vi "get_env_variable.vi"(3 "Environment Variable Name":string) -> (0 "error out":errorcluster, 1 "Value":string)   [LabVIEW 2020]
uses:
  <vilib>/Utility/config.llb/Read Key (String).vi
  <vilib>/Utility/config.llb/NI_LVConfig.lvlib
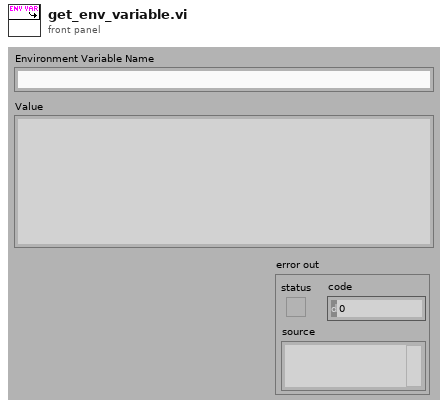
[diagram p1: front panel]
types:
  T1 = typedef "NI_LVConfig.lvlib/Config Data RefNum.ctl" = refnum<k1>
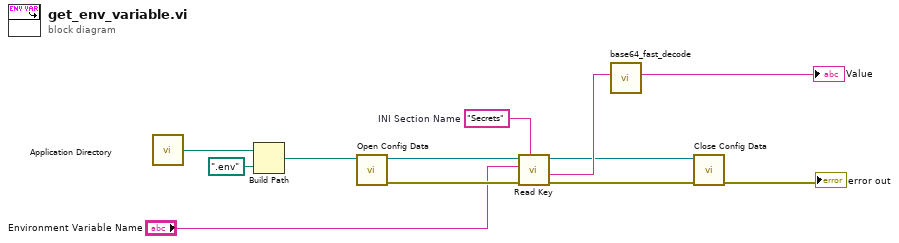
[diagram p0: block diagram]
diagram:
  w9 = "Secrets"  # INI Section Name
  n1 = call <vilib>:"Application Directory.vi"() -> ("Application Directory"=w12:path)
  n2 = Build Path(base path=w12, name or relative path=path ".env") -> (appended path=w10:path)
  n3 = call <vilib>:"Open Config Data.vi"("configuration file path"=w10) -> ("error out"=w8:errorcluster, "refnum"=w7:T1)  [unwired: 8 in, 1 out]
  n4 = call-poly <vilib>:"Read Key.vi"("section"=w9, "error in (no error)"=w8, "key"="Environment Variable Name", "refnum"=w7) -> ("error out"=w3:errorcluster, "value"=w5:string, "refnum out"=w2:T1)  [unwired: 4 in, 1 out]
  n5 = call "base64_fast_decode.vi"("string in (base64-encoded)"=w5) -> ("string out (decoded)"=→"Value":string)  [unwired: 9 in, 1 out]
  n6 = call <vilib>:"Close Config Data.vi"("error in (no error)"=w3, "refnum"=w2) -> ("error out"=→"error out":errorcluster)  [unwired: 8 in, 1 out]
